vi "Autocycle v0.3.vi"(7 "Message Queue":refnum<queue>, 8 "error in":errorcluster, 10 "All Para":cluster{"Auto Para":T1, "General Para":T2}={"Auto Para"={"Agitator Delays"=[], "TF Delays"=[], "Insertion Delays"=[], "Cutting Delays"=[], "PF Delays"=[], "Measur. Delays"=[], "Reject Delays"=[1000], "BF Delays"=[1000]}, "General Para"={"Max. Cons."=5.0, "Offset 1"=0.0, "Offset 2"=0.0, "Offset 3"=0.0, "Offset 4"=0.0}}) -> (0 "error out":errorcluster)   [LabVIEW 2017]
doc: "v0.3:\n- Added End Cycle & Stop initiated as different stops\n- Make PF & TF not run on the first iteration"
uses:
  support/Message Queue/Message Cluster.ctl
  Controls/Auto Delays.ctl
  support/Controls/General Para.ctl
  Controls/Auto Times.ctl
  Global Variables/RT GV.vi
  Global Variables/FPGA GV.vi
  <vilib>/Utility/error.llb/Error Cluster From Error Code.vi
  <vilib>/rvi/errors/niLvFpgaAdjustHostInterfaceError.vi
  support/Message Queue/Enqueue Message (Single).vi
  <vilib>/rvi/interface/nirviReadWriteControl/nirviReadWriteControl.xnode
  Controls/FPGA Ref.ctl
  NiFpgaLv.dll
  <vilib>/rvi/interface/Simulation/niFpgaSimulationCallBeginRW.vi
  support/Message Queue/Message Queue.lvlib
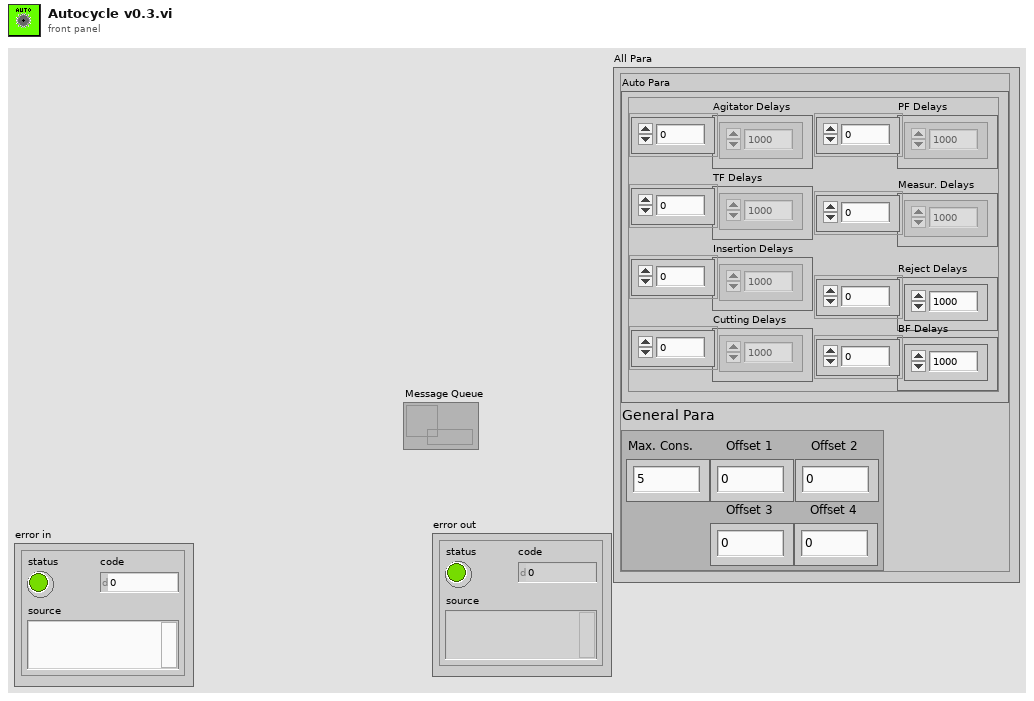
[diagram p1: front panel]
types:
  T1 = typedef "Auto Delays.ctl" = cluster{"Agitator Delays":u32[], "TF Delays":u32[], "Insertion Delays":u32[], "Cutting Delays":u32[], "PF Delays":u32[], "Measur. Delays":dbl[], "Reject Delays":u32[], "BF Delays":u32[]}
  T2 = typedef "General Para.ctl" = cluster{"Max. Cons.":dbl, "Offset 1":dbl, "Offset 2":dbl, "Offset 3":dbl, "Offset 4":dbl}
  T3 = cluster{"Tube Present":bool[], "Output Count":u32}
  T4 = typedef "FPGA Ref.ctl" = refnum<k20>
  T5 = cluster{"TL_Red":bool, "TL_Orange":bool, "TL_Green":bool, "TL_Buzzer":bool, "SOL_Index_Rotary_CW":bool, "SOL_Index_CNVR_Rotary_CCW":bool, "SOL_Index_CNVR_Stopper_Rear":bool, "SOL_Index_CNVR_Output _Separator _Rear":bool, "Bowl Feeder_ ON1":bool, "Pump_CNVR_Motor _ON":bool, "SOL_PC_Gating_CYL_Rear":bool, "SOL_Tube_Feed_Agitatator":bool, "SOL_Tube_Feed_Gating_CYL":bool, "SOL_Insertion _CYL":bool, "SOL_Insertion_Clamp_CYL":bool, "SOL_Cutting_CYL":bool, "SOL_Cutting_Clamp_CYL":bool, "SOL_Insertion_Air_Nozzle":bool, "SOL_Measurement_CYL":bool, "DO1.19":bool, "SOL_Rejection CYL_1":bool, "SOL_Rejection CYL_2":bool, "SOL_Rejection CYL_3":bool, "SOL_Rejection CYL_4":bool, "Bowl Feeder_ON2":bool, "SOL_BF_BlowerON":bool, "SOL_BF1_Track1":bool, "SOL_BF1_Track2":bool, "SOL_BF2_Track1":bool, "SOL_BF2_Track2":bool, "DO1.30":bool, "DO1.31":bool}
  T6 = typedef "Auto Times.ctl" = cluster{"Index Time":u32, "TF Time":u32, "Insertion Time":u32, "Cutting Time":u32, "PF Time":u32, "Meas. Time":u32, "Reject Time":u32}
  T7 = cluster{"Reject 1":bool, "Reject 2":bool, "Reject 3":bool, "Reject 4":bool}
  T8 = cluster{"Tube Present":bool[], "Parts Count":u32}
  T9 = cluster{"seconds since 1Jan1904":timestamp, "Auto Times":T6, "Tube Present":bool[], "Reject Pallets":cluster{"Reject 1":bool, "Reject 2":bool, "Reject 3":bool, "Reject 4":bool}, "Measurements":cluster{"1":dbl, "2":dbl, "3":dbl, "4":dbl}}
  T10 = typedef "Auto Stats.ctl" = cluster{"Time-Stamp":timestamp, "Auto Times":T6, "Measurements":cluster{"1":dbl, "2":dbl, "3":dbl, "4":dbl}, "Outputs":cluster{"Good Parts":u32, "Reject Parts":u32}, "Cycle Time":dbl, "Remarks":string}
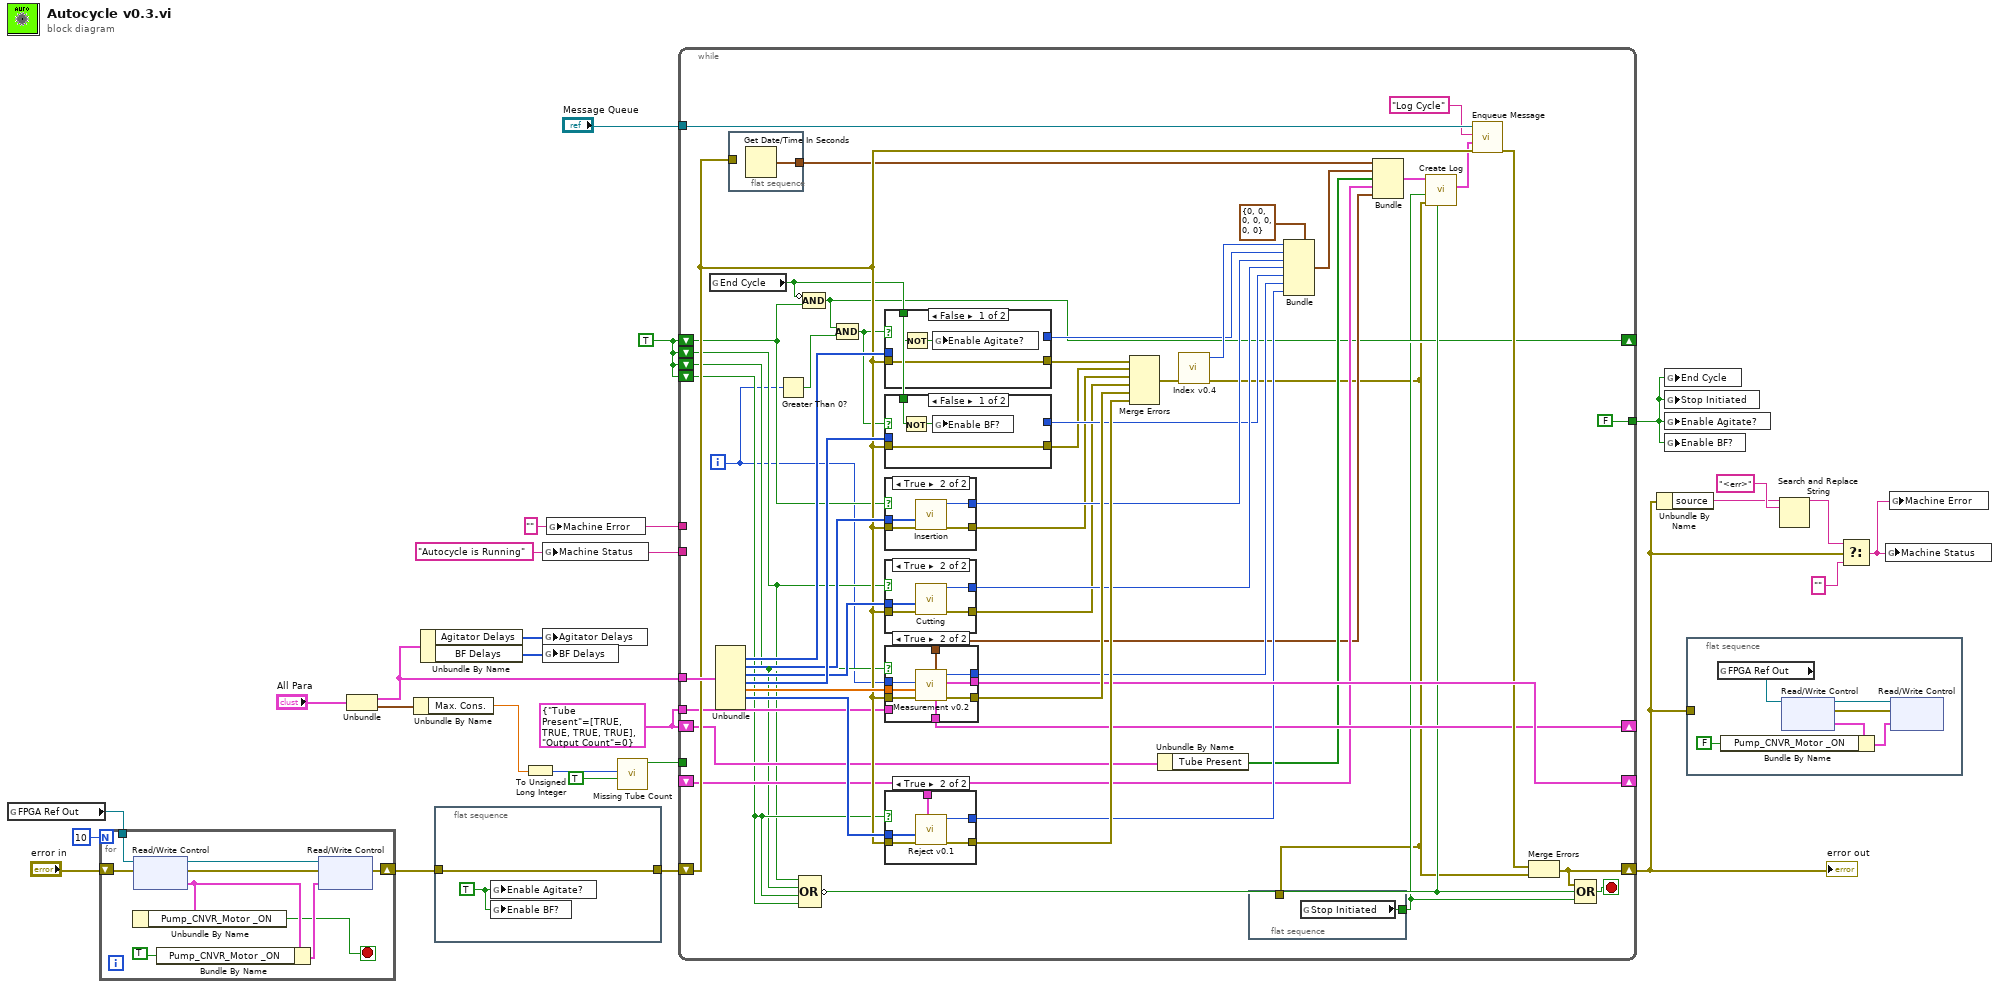
[diagram p0: block diagram]
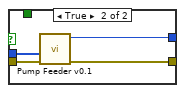
[diagram p2: hidden frame]
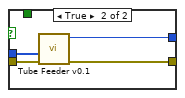
[diagram p5: hidden frame]
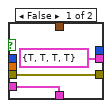
[diagram p7: hidden frame]
diagram:
  w13 = T3 {"Tube Present"=[TRUE, TRUE, TRUE, TRUE], "Output Count"=0} ("Part Count")
  w14 = "" ("Machine Error")
  w21 = "Autocycle is Running" ("Machine Status")
  w7 = TRUE
  n1 = global read "FPGA GV.vi" "FPGA Ref Out"() -> (w24:T4)
  n2 = for {
    N: 10 -> [_]
    tunnel: w24 -> [w35]
    shift-right: [w29] -> w10
    shift-left: "error in" -> [w30]
    stop <- w27 stop-if-true
    n3 = xnode "Read/Write Control"("FPGA VI Reference In"=w35, "error in"=w30) -> ("FPGA VI Reference Out"=w31:T4, "error out"=w32:errorcluster, "DO 1"=w28:T5)
    n4 = Unbundle By Name(w28) -> ("Pump_CNVR_Motor _ON"=w27:bool)
    n5 = Bundle By Name(cluster=w28, "Pump_CNVR_Motor _ON"=TRUE) -> (w34:T5)
    n6 = xnode "Read/Write Control"("FPGA VI Reference In"=w31, "error in"=w32, "DO 1"=w34) -> ("error out"=w29:errorcluster)  [unwired: 1 out]
  }
  n7 = Unbundle("All Para") -> ("Auto Para"=w4:T1, "General Para"=w3:T2)
  n8 = Unbundle By Name(w3) -> ("Max. Cons."=w2:dbl)
  n9 = Unbundle By Name(w4) -> ("Agitator Delays"=w26:u32[], "BF Delays"=w25:u32[])
  n10 = flat-sequence {
    tunnel: [w37] -> w9
    tunnel: w10 -> [w37]
    frame #0 {
      w36 = TRUE ("Enable Agitate?")
      n11 = global write "RT GV.vi" "Enable Agitate?"(w36) -> ()
      n12 = global write "RT GV.vi" "Enable BF?"(w36) -> ()
    }
  }
  n13 = To Unsigned Long Integer(number=w2) -> (unsigned 32bit integer=w1:u32)
  n14 = global write "RT GV.vi" "Machine Status"(w21) -> ()
  n15 = global write "RT GV.vi" "Agitator Delays"(w26) -> ()
  n16 = global write "RT GV.vi" "BF Delays"(w25) -> ()
  n17 = global write "RT GV.vi" "Machine Error"(w14) -> ()
  n18 = call "Missing Tube Count.vi"("ResetMT?"=TRUE, "Max Successive"=w1) -> ("Boolean"=w11:bool)  [unwired: 9 in]
  n19 = while {
    tunnel: w4 -> [w85]
    shift-right: [w61] -> w19
    shift-left: w9 -> [w63]
    shift-right: [w79] -> _
    shift-left: _ -> [w52]
    shift-right: [w43] -> _
    shift-left: w7 -> [w44]
    shift-left: w7 -> [w45]
    shift-left: w7 -> [w46]
    shift-left: w7 -> [w47]
    tunnel: "Message Queue" -> [w69]
    tunnel: [FALSE] -> w6
    tunnel: w21 -> [_]
    tunnel: w14 -> [_]
    shift-right: [w55] -> _
    shift-left: w13 -> [w54]
    tunnel: w13 -> [w56]
    tunnel: w11 -> [_]
    i -> [w39]
    stop <- w78 stop-if-true
    n20 = global read "RT GV.vi" "End Cycle"() -> (w48:bool)
    n21 = Unbundle(w85) -> ("TF Delays"=w88:u32[], "Insertion Delays"=w87:u32[], "Cutting Delays"=w86:u32[], "PF Delays"=w89:u32[], "Measur. Delays"=w83:dbl[], "Reject Delays"=w81:u32[])  [unwired: 2 out]
    n22 = flat-sequence {
      tunnel: w63 -> [_]
      tunnel: [w91] -> w58
      frame #0 {
        n23 = Get Date/Time In Seconds() -> (seconds since 1Jan1904=w91:timestamp)
      }
    }
    n24 = Greater Than 0?(x=w39) -> (x > 0?=w41:bool)
    n25 = Compound Arithmetic op=OR(w45, w46, w47, w47) -> (invert w50:bool)
    n26 = Compound Arithmetic op=AND(invert w48, w44) -> (w43:bool)
    n27 = Compound Arithmetic op=AND(w43, w41) -> (w42:bool)
    n28 = case shown="False" w42 {
      tunnel: w63 -> [w111 w115]
      tunnel: [w111 w114] -> w84
      tunnel: w88 -> [_ w113]
      tunnel: [_ w112] -> w76
      tunnel: w48 -> [w110 _]
      frame False {
        n29 = Not(x=w110) -> (.not. x?=w109:bool)
        n30 = global write "RT GV.vi" "Enable Agitate?"(w109) -> ()
      }
      frame True {
        n31 = call "Tube Feeder v0.1.vi"("error in (no error)"=w115, "TF Para"=w113) -> ("error out"=w114:errorcluster, "TF Time"=w112:u32)  [unwired: 8 in]
      }
    }
    n32 = case shown="False" w42 {
      tunnel: w63 -> [w94 w98]
      tunnel: [w94 w97] -> w65
      tunnel: w89 -> [_ w96]
      tunnel: [_ w95] -> w73
      tunnel: w48 -> [w93 _]
      frame False {
        n33 = Not(x=w93) -> (.not. x?=w92:bool)
        n34 = global write "RT GV.vi" "Enable BF?"(w92) -> ()
      }
      frame True {
        n35 = call "Pump Feeder v0.1.vi"("error in (no error)"=w98, "TF Delays"=w96) -> ("error out"=w97:errorcluster, "PF Time"=w95:u32)  [unwired: 8 in]
      }
    }
    n36 = case shown="True" w44 {
      tunnel: w63 -> [w104 w108]
      tunnel: [w104 w107] -> w66
      tunnel: w87 -> [_ w106]
      tunnel: [_ w105] -> w75
      frame False {
      }
      frame True {
        n37 = call "Insertion.vi"("error in (no error)"=w108, "Insertion Delays"=w106) -> ("error out"=w107:errorcluster, "Insertion Time"=w105:u32)  [unwired: 7 in, 1 out]
      }
    }
    n38 = case shown="True" w45 {
      tunnel: w63 -> [w99 w103]
      tunnel: [w99 w102] -> w67
      tunnel: w86 -> [_ w101]
      tunnel: [_ w100] -> w74
      frame False {
      }
      frame True {
        n39 = call "Cutting.vi"("error in (no error)"=w103, "Cutting Delays"=w101) -> ("error out"=w102:errorcluster, "Cutting Time"=w100:u32)  [unwired: 8 in]
      }
    }
    n40 = case shown="True" w46 {
      tunnel: w63 -> [w124 w132]
      tunnel: [w124 w131] -> w82
      tunnel: w83 -> [_ w130]
      tunnel: [_ w129] -> w72
      tunnel: [_ w128] -> w51
      tunnel: [T7 {"Reject 1"=TRUE, "Reject 2"=TRUE, "Reject 3"=TRUE, "Reject 4"=TRUE} ("Reject Pallets") w127] -> w79
      tunnel: [w122 w126] -> w55
      tunnel: w56 -> [w122 _]
      tunnel: w39 -> [_ w125]
      frame False {
      }
      frame True {
        n41 = call "Measurement v0.2.vi"("error in (no error)"=w132, "TF Delays"=w130, "Loop Count"=w125) -> ("error out"=w131:errorcluster, "Reject Pallets"=w127:T7, "PF Time"=w129:u32, "Part Count"=w126:T8, "Measurements"=w128:cluster{"1":dbl, "2":dbl, "3":dbl, "4":dbl})  [unwired: 4 in]
      }
    }
    n42 = case shown="True" w47 {
      tunnel: w63 -> [w116 w121]
      tunnel: [w116 w120] -> w80
      tunnel: w81 -> [_ w119]
      tunnel: [_ w118] -> w71
      tunnel: w52 -> [_ w117]
      frame False {
      }
      frame True {
        n43 = call "Reject v0.1.vi"("Reject Pallets"=w117, "error in (no error)"=w121, "TF Delays"=w119) -> ("error out"=w120:errorcluster, "PF Time"=w118:u32)  [unwired: 7 in]
      }
    }
    n44 = Merge Errors(w84, w65, w66, w67, w82, w80) -> (w62:errorcluster)
    n45 = Unbundle By Name(w54) -> ("Tube Present"=w53:bool[])
    n46 = call "Index v0.4.vi"("error in (no error)"=w62) -> ("error out"=w38:errorcluster, "Index Time"=w77:u32)  [unwired: 7 in, 2 out]
    n47 = flat-sequence {
      tunnel: [w90] -> w40
      tunnel: w38 -> [_]
      frame #0 {
        n48 = global read "RT GV.vi" "Stop Initiated"() -> (w90:bool)
      }
    }
    n49 = Bundle(cluster=T6 {"Index Time"=0, "TF Time"=0, "Insertion Time"=0, "Cutting Time"=0, "PF Time"=0, "Meas. Time"=0, "Reject Time"=0} ("Auto Times"), "Index Time"=w77, "TF Time"=w76, "Insertion Time"=w75, "Cutting Time"=w74, "PF Time"=w73, "Meas. Time"=w72, "Reject Time"=w71) -> (w57:T6)
    n50 = Bundle("seconds since 1Jan1904"=w58, "Auto Times"=w57, "Tube Present"=w53, "Reject Pallets"=w52, "Measurements"=w51) -> (w49:T9)  [unwired: 1 in]
    n51 = call "Create Log.vi"("End Cycle?"=w50, "Error in"=w38, "Stop Initiated?"=w40, "Log Input Data"=w49) -> ("Auto Stats"=w59:T10)  [unwired: 7 in]
    n52 = call-poly "Enqueue Message.vi"("error in (no error)"=w63, "Message Data"=w59, "Message"="Log Cycle", "Message Queue"=w69) -> ("error out"=w60:errorcluster)  [unwired: 6 in, 1 out]
    n53 = Merge Errors(w60, w38) -> (w61:errorcluster)
    n54 = Compound Arithmetic op=OR(w61, w50, w40) -> (w78:bool)
  }
  "error out" <- w19
  n55 = Unbundle By Name(w19) -> ("source"=w17:string)
  n56 = global write "RT GV.vi" "End Cycle"(w6) -> ()
  n57 = global write "RT GV.vi" "Stop Initiated"(w6) -> ()
  n58 = global write "RT GV.vi" "Enable Agitate?"(w6) -> ()
  n59 = global write "RT GV.vi" "Enable BF?"(w6) -> ()
  n60 = flat-sequence {
    tunnel: w19 -> [_]
    frame #0 {
      n61 = global read "FPGA GV.vi" "FPGA Ref Out"() -> (w133:T4)
      n62 = xnode "Read/Write Control"("FPGA VI Reference In"=w133) -> ("FPGA VI Reference Out"=w138:T4, "error out"=w137:errorcluster, "DO 1"=w135:T5)  [unwired: 1 in]
      n63 = Bundle By Name(cluster=w135, "Pump_CNVR_Motor _ON"=FALSE) -> (w136:T5)
      n64 = xnode "Read/Write Control"("FPGA VI Reference In"=w138, "error in"=w137, "DO 1"=w136) -> ()  [unwired: 2 out]
    }
  }
  n65 = Search and Replace String(input string=w17, search string="<err>") -> (result string=w16:string)  [unwired: 6 in, 3 out]
  n66 = Select(t=w16, s=w19, f="" ("Machine Status")) -> (s? t:f=w15:string)
  n67 = global write "RT GV.vi" "Machine Status"(w15) -> ()
  n68 = global write "RT GV.vi" "Machine Error"(w15) -> ()
